vi "initialize_devices.vi"(0 "AWG VISA Name":refnum<visa-resource-name>="AWG5014C", 5 "Reference Name":string="Reference Wave", 7 "Reference Amplitude":dbl=0.4081632653061224, 9 "Cant. Freq":dbl=18488.0, 11 "LIA VISA Name":refnum<visa-resource-name>="SR865", 13 "no. periods":i32=1) -> (3 "time to wait":dbl, 4 "AWG VISA out":refnum<visa-resource-name>="AWG5014C", 6 "error out":errorcluster, 8 "config out":string, 10 "error out 2":errorcluster, 15 "LIA VISA out":refnum<visa-resource-name>="SR865")   [LabVIEW 2018]
uses:
  <instrlib>/Tektronix AWG 5000 7000 Series/Public/Configure/Channel/Assign Output Waveform (From Waveform List).vi
  <instrlib>/Stanford Research SR865/Stanford Research SR865.lvlib
  <instrlib>/Tektronix AWG 5000 7000 Series/Tektronix AWG 5000 7000 Series.lvlib
panel:
  in  "Wait time (ms)":dbl
  in  "Sensitivity (0: 1 V [uA])":i32(ring)=6 items=["Auto Scale"=-1, "1 V [uA]"=0, "500 mV [nA] "=1, "200 mV [nA]"=2, "100 mV [nA] "=3, "50 mV [nA]"=4, "20 mV [nA] "=5, "10 mV [nA] "=6, "5 mV [nA]"=7, "2 mV [nA] "=8, "1 mV [nA] "=9, "500 uV [pA] "=10, "200 uV [pA]"=11, "100 uV [pA] "=12, "50 uV [pA]"=13, "20 uV [pA]"=14, "10 uV [pA]"=15, "5 uV [pA]"=16, "2 uV [pA]"=17, "1 uV [pA]"=18, "500 nV [fA]"=19, "200 nV [fA]"=20, "100 nV [fA]"=21, "50 nV [fA]"=22, "20 nV [fA]"=23, "10 nV [fA]"=24, "5 nV [fA]"=25, "2 nV [fA]"=26, "1 nV [fA]"=27]
  in  "Voltage Input Range (0: 1V)":i32(ring)=2 items=["Auto Range"=-1, "1V"=0, "300mV"=1, "100mV"=2, "30mV"=3, "10mV"=4]
  in  "Filter Slope (0: 6 dB/oct)":u16(ring)=2 items=["6 dB/oct", "12 dB/oct", "18 dB/oct", "24 dB/oct"]
  in  "Time Constant (10: 100 ms)":u16(ring)=9 items=["1 us", "3 us", "10 us", "30 us", "100 us", "300 us", "1 ms", "3 ms", "10 ms", "30 ms", "100 ms", "300 ms", "1 s", "3 s", "10 s", "30 s", "100 s", "300 s", "1 ks", "3 ks", "10 ks", "30 ks"]
  in  "Reset (False)":bool=TRUE
  # "V"
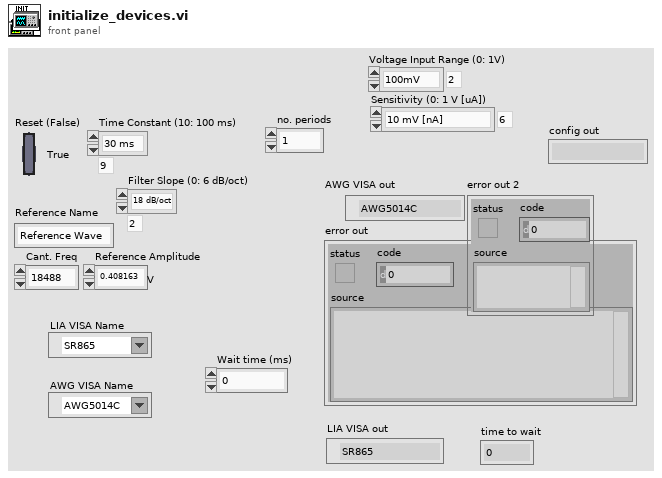
[diagram p1: front panel]
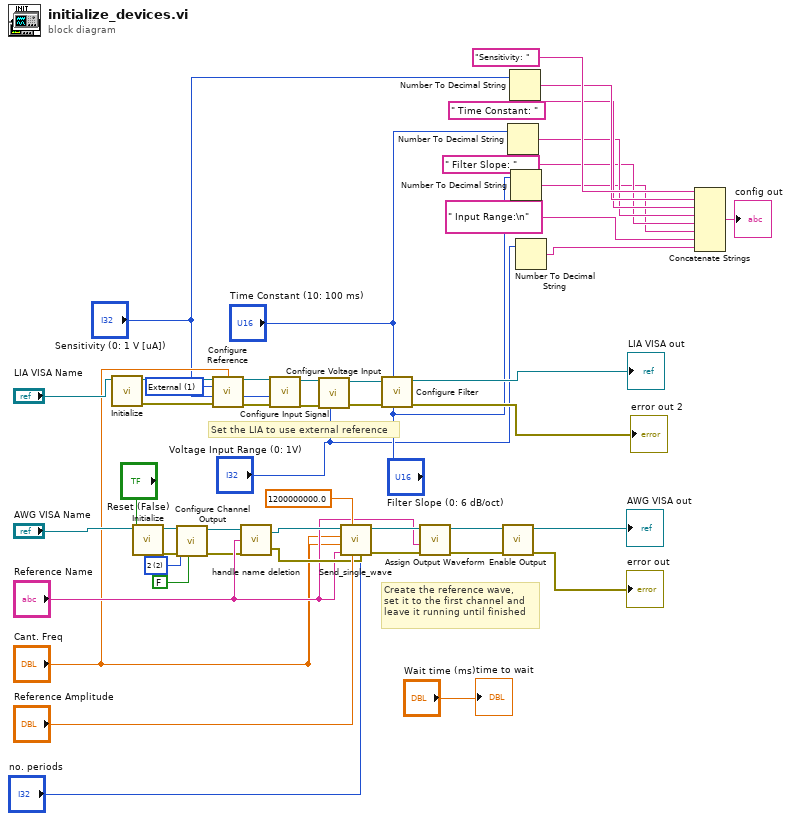
[diagram p0: block diagram]
diagram:
  w16 = u16 2 items=["1"=1, "2"=2, "3"=3, "4"=4] ("Channel Name (1)")
  w35 = 1 items=["Internal", "External", "Dual", "Chop"] ("Reference Source (0: Internal)")
  # "Set the LIA to use external reference"
  # "Create the reference wave,\nset it to the first channel and\nleave it running until finished"
  n1 = call <instrlib>:"Initialize.vi"("VISA resource name"="LIA VISA Name") -> ("error out"=w37:errorcluster, "VISA resource name out"=w39:refnum<visa-resource-name>)  [unwired: 9 in]
  n2 = call <instrlib>:"Initialize.vi"("Reset (False)"="Reset (False)", "VISA resource name"="AWG VISA Name") -> ("error out"=w17:errorcluster, "VISA resource name out"=w20:refnum<visa-resource-name>)  [unwired: 8 in]
  n3 = call <instrlib>:"Configure Channel Output.vi"("Enable Direct Output (F : Disable)"=FALSE, "error in (no error)"=w17, "Channel Name (1)"=w16, "VISA resource name"=w20) -> ("error out"=w18:errorcluster, "VISA resource name out"=w19:refnum<visa-resource-name>)  [unwired: 6 in]
  n4 = call <instrlib>:"Configure Reference.vi"("VISA resource name"=w39, "Internal Reference Frequency (100000Hz)"="Cant. Freq", "Reference Source (0: Internal)"=w35, "error in (no error)"=w37) -> ("VISA resource name out"=w38:refnum<visa-resource-name>, "error out"=w36:errorcluster)  [unwired: 10 in]
  n5 = call "handle name deletion.vi"("error in (no error)"=w18, "String"="Reference Name", "VISA resource name"=w19) -> ("error out"=w31:errorcluster, "VISA resource name out"=w32:refnum<visa-resource-name>)
  n6 = call <instrlib>:"Configure Input Signal.vi"("error in (no error)"=w36, "Sensitivity (0: 1 V [uA])"="Sensitivity (0: 1 V [uA])", "VISA resource name"=w38) -> ("error out"=w22:errorcluster, "VISA resource name out"=w25:refnum<visa-resource-name>)  [unwired: 7 in]
  n7 = call <instrlib>:"Configure Voltage Input.vi"("Voltage Input Range (0: 1V)"="Voltage Input Range (0: 1V)", "error in (no error)"=w22, "VISA resource name"=w25) -> ("error out"=w23:errorcluster, "VISA resource name out"=w24:refnum<visa-resource-name>)  [unwired: 7 in]
  n8 = call "Send_single_wave.vi"("error in (no error)"=w31, "no. periods"="no. periods", "Amplitude"="Reference Amplitude", "Max sample rate"=1200000000.0, "Name"="Reference Name", "Cant. Freq"="Cant. Freq", "Frequency"="Cant. Freq", "VISA resource name"=w32) -> ("error out"=w45:errorcluster, "VISA resource name out"=w44:refnum<visa-resource-name>)  [unwired: 2 in]
  n9 = call <instrlib>:"Configure Filter.vi"("Filter Slope (0: 6 dB/oct)"="Filter Slope (0: 6 dB/oct)", "Time Constant (10: 100 ms)"="Time Constant (10: 100 ms)", "error in (no error)"=w23, "VISA resource name"=w24) -> ("error out"=→"error out 2":errorcluster, "VISA resource name out"=→"LIA VISA out":refnum<visa-resource-name>)  [unwired: 6 in]
  n10 = call-poly <instrlib>:"Assign Output Waveform.vi"("error in (no error)"=w45, "Waveform"="Reference Name", "VISA resource name"=w44) -> ("error out"=w42:errorcluster, "VISA resource name out"=w41:refnum<visa-resource-name>)  [unwired: 7 in]
  n11 = call <instrlib>:"Enable Output.vi"("error in (no error)"=w42, "VISA resource name"=w41) -> ("error out"=→"error out":errorcluster, "VISA resource name out"=→"AWG VISA out":refnum<visa-resource-name>)  [unwired: 8 in]
  n12 = Number To Decimal String(number="Time Constant (10: 100 ms)") -> (decimal integer string=w8:string)  [unwired: 1 in]
  n13 = Number To Decimal String(number="Sensitivity (0: 1 V [uA])") -> (decimal integer string=w11:string)  [unwired: 1 in]
  n14 = Number To Decimal String(number="Filter Slope (0: 6 dB/oct)") -> (decimal integer string=w5:string)  [unwired: 1 in]
  n15 = Number To Decimal String(number="Voltage Input Range (0: 1V)") -> (decimal integer string=w3:string)  [unwired: 1 in]
  n16 = Concatenate Strings("Sensitivity: ", w11, " Time Constant: ", w8, " Filter Slope: ", w5, " Input Range:\n", w3) -> (→"config out":string)
  "time to wait" <- "Wait time (ms)"
